vi "GetIPMy.vi"() -> (1 "IP address":string)   [LabVIEW 2010]
panel:
  out "before substring":string
  out "standard output":string
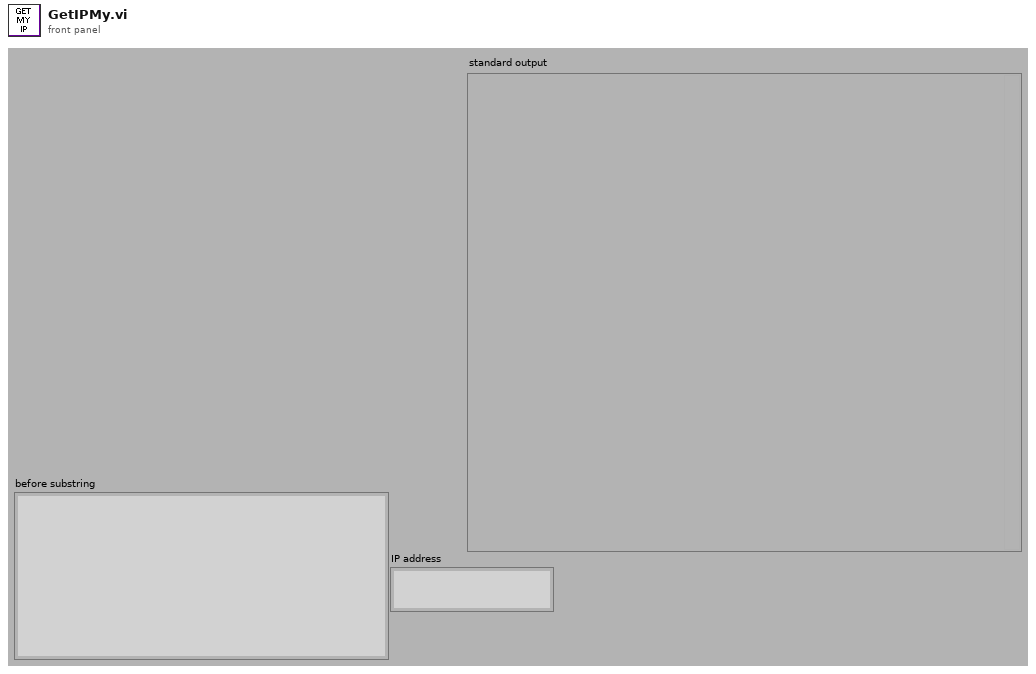
[diagram p1: front panel]
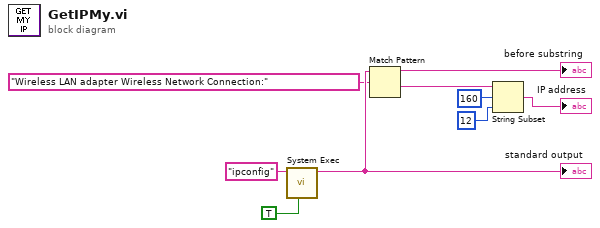
[diagram p0: block diagram]
diagram:
  n1 = call <vilib>:"System Exec.vi"("run minimized? (F)"=TRUE, "command line"="ipconfig") -> ("standard output"=w7:string)  [unwired: 6 in, 3 out]
  "standard output" <- w7
  n2 = Match Pattern(string=w7, regular expression="Wireless LAN adapter Wireless Network Connection:") -> (before substring=→"before substring":string, after substring=w1:string)  [unwired: 1 in, 2 out]
  n3 = String Subset(string=w1, offset (0)=160, length (rest)=12 ("length (rest)")) -> (substring=→"IP address":string)
